vi "bmd101Parser_v2.vi"() -> ()   [LabVIEW 2016]
uses:
  C:/Program Files/National Instruments/LabVIEW 2016/examples/Instrument IO/Serial/support/Serial - Settings.ctl
  State.ctl
  <vilib>/Instr/_visa.llb/VISA Configure Serial Port (Instr).vi
panel:
  out "subarray":u8[](array[numeric])
  out "16bit integer":i16
  in  "Stop":bool
  out "unsigned byte array":u8[](array[numeric]) format="%x"
  in  "byte count":u32=1
  out "Array":u8[](array[numeric]) format="%x"
  out "error IO":errorcluster={"status"=FALSE, "code"=-1074118647, "source"=""}
  out "ECG":i16(graph)
  in  "Serial Settings":T1={"baud rate"=57600, "data bits"=8, "parity"=enum."None", "stop bits"=10, "flow control"=0} {"flow control" items=["None"=0, "XON/XOFF"=1, "RTS/CTS"=2, "DTR/DSR"=4]; "stop bits" items=["1.0"=10, "1.5"=15, "2.0"=20]; "data bits" min=5 max=8 step=1; "baud rate" items=["75"=75, "110"=110, "134"=134, "150"=150, "300"=300, "600"=600, "1200"=1200, "1800"=1800, "2400"=2400, "4800"=4800, "7200"=7200, "9600"=9600, "14400"=14400, "19200"=19200, "28800"=28800, "38400"=38400, "56000"=56000, "57600"=57600, "115200"=115200, "128000"=128000, "230400"=230400]}
  in  "VISA resource name":refnum<visa-resource-name>="bmd101"
  out "Packets Recieved":i32
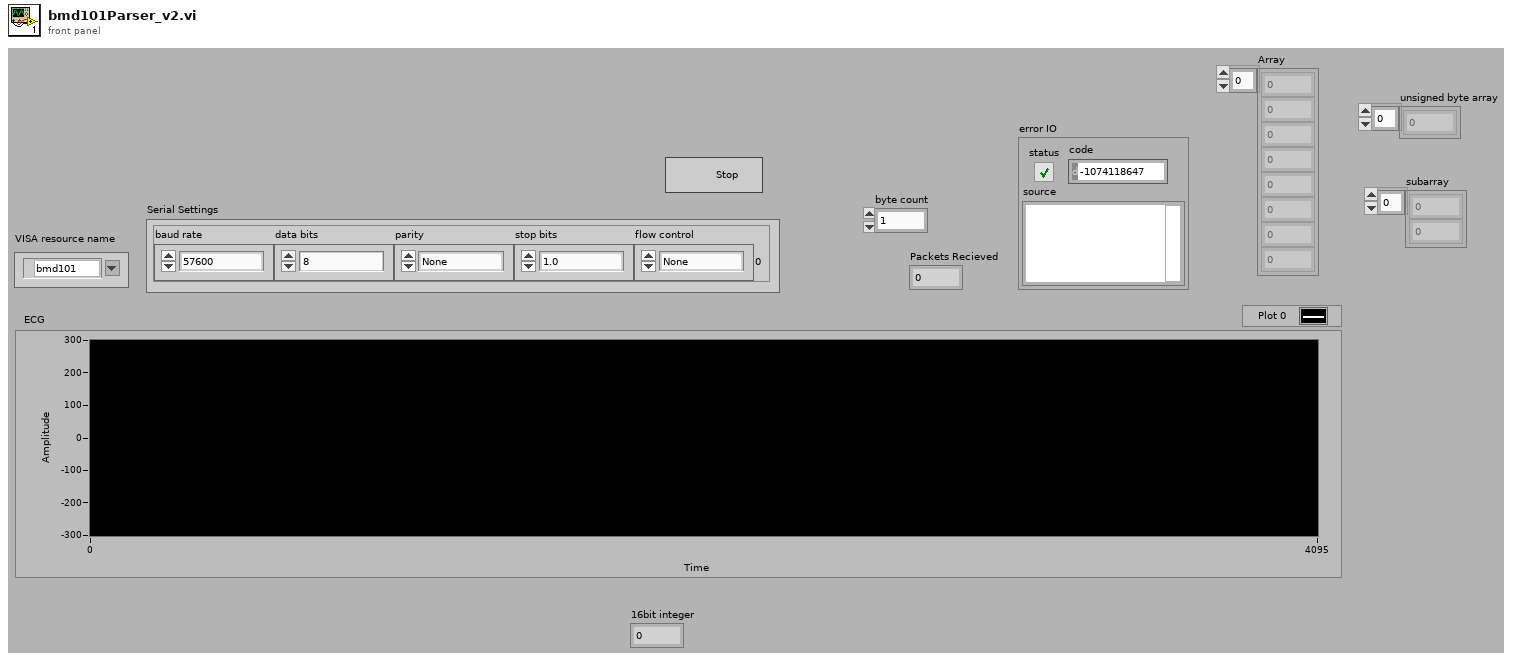
[diagram p1: front panel]
types:
  T1 = typedef "Serial - Settings.ctl" = cluster{"baud rate":u32, "data bits":u16, "parity":enum16{"None", "Odd", "Even", "Mark", "Space"}, "stop bits":u16, "flow control":u16}
  T2 = typedef "State.ctl" = enum16{"Initialize", "get byte", "check", "packet received", "packet approved"}
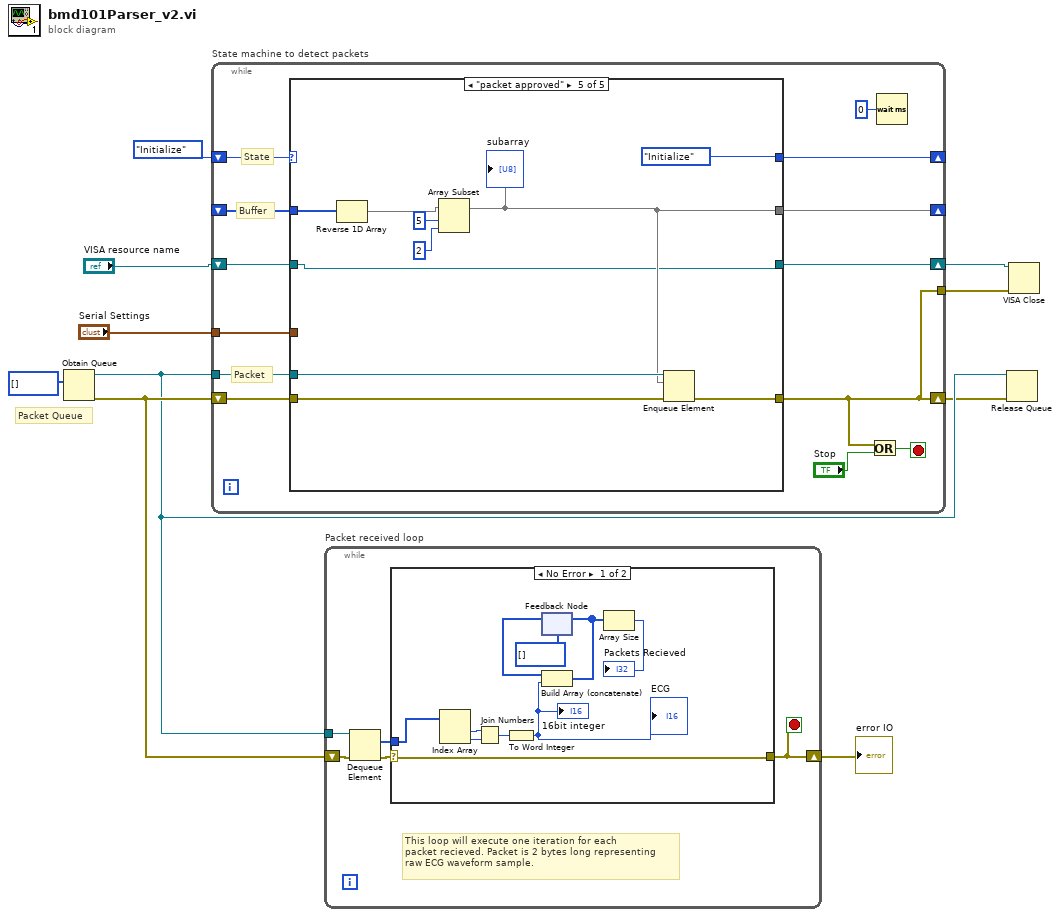
[diagram p0: block diagram]
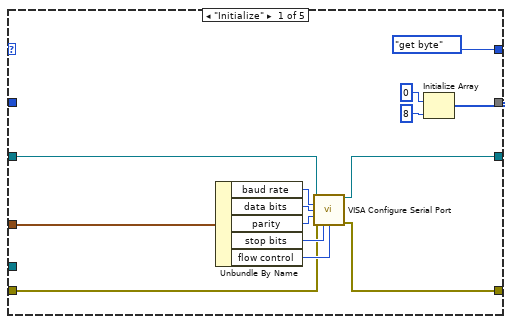
[diagram p3: hidden frame]
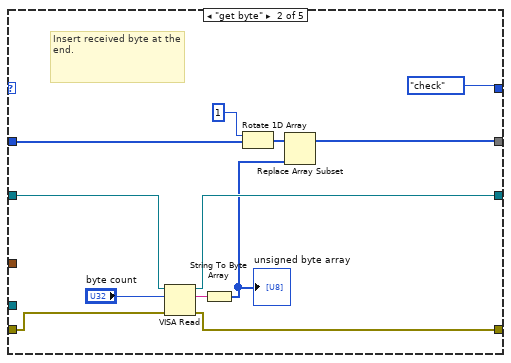
[diagram p4: hidden frame]
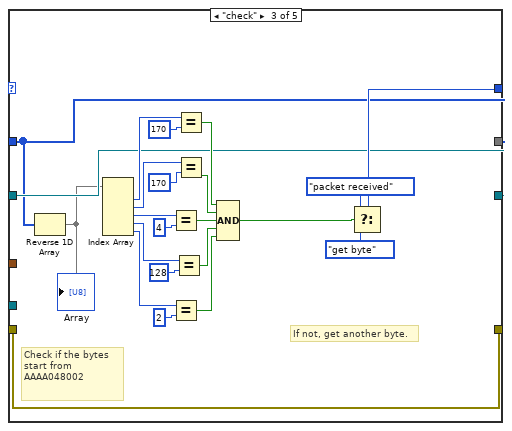
[diagram p5: hidden frame]
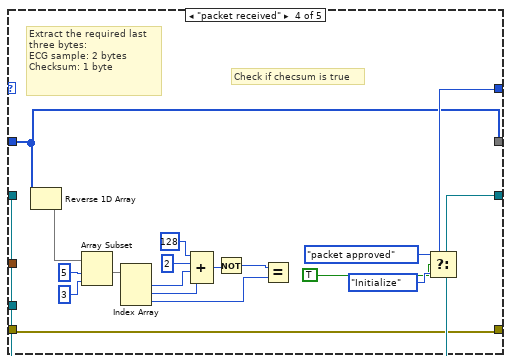
[diagram p6: hidden frame]
diagram:
  # "Packet Queue"
  n1 = Obtain Queue(element data type=u8[] []) -> (queue out=w7:refnum<queue>, error out=w8:errorcluster)  [unwired: 4 in, 1 out]
  n2 = while "State machine to detect packets" {
    shift-right: [w14] -> w2
    shift-left: w8 -> [w20]
    shift-right: [w23] -> _
    shift-left: State."Initialize" ("State") -> [w22]
    shift-right: [w19] -> _
    shift-left: _ -> [w21]
    tunnel: w7 -> [w18]
    shift-right: [w17] -> w3
    shift-left: "VISA resource name" -> [w16]
    tunnel: "Serial Settings" -> [w15]
    tunnel: [w14] -> w1
    stop <- w12 stop-if-true
    # "State"
    # "Buffer"
    # "Packet"
    n3 = case shown="\"packet approved\"" w22 {
      tunnel: [w34 w47 w51 w74 w94] -> w19
      tunnel: [State."get byte" ("State") State."check" ("f") w71 w80 State."Initialize" ("State")] -> w23
      tunnel: w21 -> [_ w39 w51 w74 w92]
      tunnel: w20 -> [w28 w43 w72 w81 w96]
      tunnel: [w27 w42 w72 w81 w95] -> w14
      tunnel: w18 -> [_ _ _ _ w97]
      tunnel: [w26 w45 w52 w88 w93] -> w17
      tunnel: w16 -> [w25 w46 w52 w88 w93]
      tunnel: w15 -> [w24 _ _ _ _]
      frame "Initialize" {
        n4 = Unbundle By Name(w24) -> ("baud rate"=w33:u32, "data bits"=w32:u16, "parity"=w31:enum16{"None", "Odd", "Even", "Mark", "Space"}, "stop bits"=w30:u16, "flow control"=w29:u16)
        n5 = call-poly "VISA Configure Serial Port"("VISA resource name"=w25, "baud rate (9600)"=w33, "data bits (8)"=w32, "parity (0:none)"=w31, "error in (no error)"=w28, "stop bits (10: 1 bit)"=w30, "flow control (0:none)"=w29) -> ("VISA resource name out"=w26:refnum<visa-resource-name>, "error out"=w27:errorcluster)  [unwired: 3 in, 4 out]
        n6 = Initialize Array(u8 0, 8 ("dimension size")) -> (w34:u8[])
      }
      frame "get byte" {
        # "Insert received byte at the end."
        n7 = VISA Read(VISA resource name=w46, byte count="byte count", error in (no error)=w43) -> (VISA resource name out=w45:refnum<visa-resource-name>, read buffer=w41:string, error out=w42:errorcluster)  [unwired: 1 out]
        n8 = String To Byte Array(string=w41) -> (unsigned byte array=w40:u8[])
        "unsigned byte array" <- w40
        n9 = Rotate 1D Array(1:w39, 2:1) -> (0:w48:u8[])
        n10 = Replace Array Subset(array=w48, new element=w40) -> (w47:u8[])  [unwired: 1 in]
      }
      frame "check" {
        # "If not, get another byte."
        # "Check if the bytes start from AAAA048002"
        n11 = Reverse 1D Array(array=w51) -> (reversed array=w50:u8[])
        "Array" <- w50
        n12 = Index Array(array=w50) -> (element #1=w58:u8, element #2=w57:u8, element #3=w56:u8, element #4=w55:u8, element #5=w54:u8)  [unwired: 5 in]
        n13 = Equal?(x=w56, y=u8 4 ("element")) -> (x = y?=w61:bool)
        n14 = Equal?(x=w54, y=u8 2 ("element")) -> (x = y?=w59:bool)
        n15 = Equal?(x=w55, y=u8 128 ("element")) -> (x = y?=w60:bool)
        n16 = Equal?(x=w58, y=u8 170 ("element")) -> (x = y?=w63:bool)
        n17 = Equal?(x=w57, y=u8 170 ("element")) -> (x = y?=w62:bool)
        n18 = Compound Arithmetic op=AND(w63, w62, w61, w60, w59) -> (w53:bool)
        n19 = Select(t=State."packet received" ("f"), s=w53, f=State."get byte") -> (s? t:f=w71:T2)
      }
      frame "packet received" {
        # "Check if checsum is true"
        # "Extract the required last three bytes: \nECG sample: 2 bytes\nChecksum: 1 byte"
        n20 = Reverse 1D Array(array=w74) -> (reversed array=w73:u8[])
        n21 = Array Subset(array=w73, index=5, length=3 ("index")) -> (w87:u8[])
        n22 = Index Array(array=w87) -> (element #1=w82:u8, element #2=w83:u8, element #3=w84:u8)  [unwired: 3 in]
        n23 = Compound Arithmetic op=ADD(u8 128 ("element"), u8 2 ("element"), w82, w83) -> (w77:u8)
        n24 = Not(x=w77) -> (.not. x?=w76:u8)
        n25 = Equal?(x=w76, y=w84) -> ()  [unwired: 1 out]
        n26 = Select(t=State."packet approved" ("State"), s=TRUE, f=State."Initialize" ("State")) -> (s? t:f=w80:T2)
      }
      frame "packet approved" {
        n27 = Reverse 1D Array(array=w92) -> (reversed array=w91:u8[])
        n28 = Array Subset(array=w91, index=5, length=2 ("index")) -> (w94:u8[])
        "subarray" <- w94
        n29 = Enqueue Element(queue=w97, element=w94, error in (no error)=w96) -> (error out=w95:errorcluster)  [unwired: 1 in, 2 out]
      }
    }
    n30 = Or(x=w14, y="Stop") -> (x .or. y?=w12:bool)
    n31 = Wait (ms)(milliseconds to wait=u32 0) -> ()  [unwired: 1 out]
  }
  n32 = while "Packet received loop" {
    shift-right: [w101] -> w4
    shift-left: w8 -> [w105]
    tunnel: w7 -> [w104]
    stop <- w101 stop-if-true
    # "This loop will execute one iteration for each\npacket recieved. Packet is 2 bytes long representing \nraw ECG waveform sample."
    n33 = Dequeue Element(queue=w104, error in (no error)=w105) -> (element=w103:u8[], error out=w102:errorcluster)  [unwired: 1 in, 2 out]
    n34 = case shown="No Error" w102 {
      selector: w102 -> [w115 w116]
      tunnel: w103 -> [w114 _]
      tunnel: [w115 w116] -> w101
      frame No Error {
        n35 = Index Array(array=w114) -> (element #1=w113:u8, element #2=w112:u8)  [unwired: 2 in]
        n36 = Join Numbers(hi=w113, lo=w112) -> ((hi.lo)=w111:u16)
        n37 = To Word Integer(number=w111) -> (16bit integer=w106:i16)
        "ECG" <- w106
        "16bit integer" <- w106
        n38 = feedback #1(i32[] []) -> (w109:i32[])
        n39 = Build Array (concatenate)(w109, w106) -> (w108:i32[])
        n40 = feedback-in #1(w108) -> ()
        n41 = Array Size(array=w108) -> (size(s)=→"Packets Recieved":i32)
      }
      frame Error {
      }
    }
  }
  "error IO" <- w4
  n42 = Release Queue(queue=w7, error in (no error)=w2) -> ()  [unwired: 1 in, 3 out]
  n43 = VISA Close(VISA resource name=w3, error in (no error)=w1) -> ()  [unwired: 1 out]
